vi "execute_initial_value_policy.vi"(8 "error in (no error)":errorcluster, 9 "Last Publish Time":timestamp, 10 "Last Topic Value":variant, 11 "ValueChangeSubscription In":refnum<class "ValueChangeSubscription.lvclass">) -> (0 "error out":errorcluster, 3 "ValueChangeSubscription Out":refnum<class "ValueChangeSubscription.lvclass">)   [LabVIEW 2017, in "SubscriptionPolicy.lvlib" / "ValueChangeSubscription.lvclass"]
uses:
  ValueChangeSubscription.lvclass
  ValueChangeSubscription.lvclass/ValueChangeSubscription.ctl
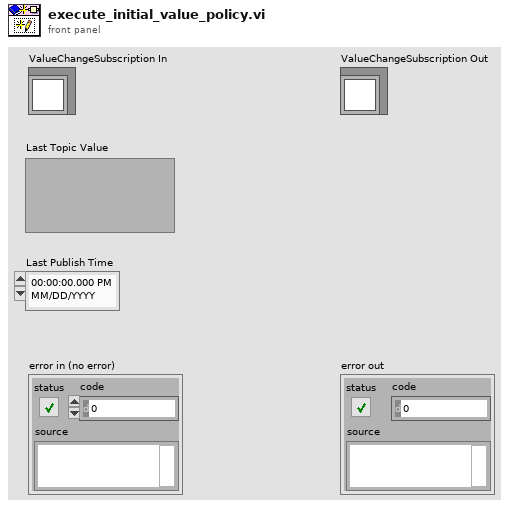
[diagram p1: front panel]
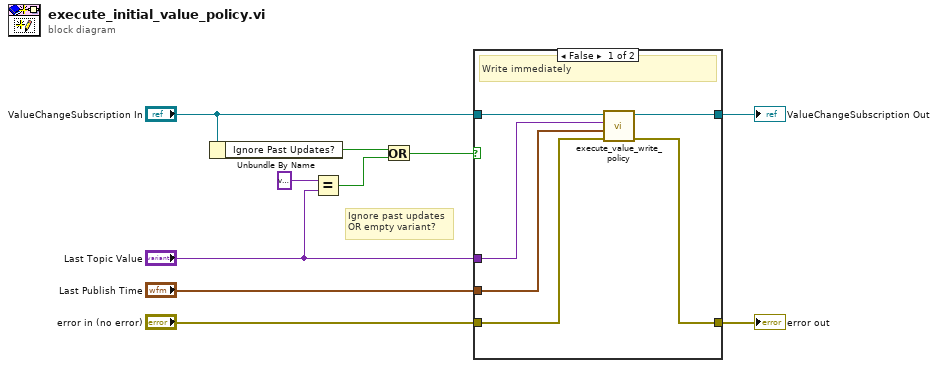
[diagram p0: block diagram]
diagram:
  # "Ignore past updates\nOR empty variant?"
  n1 = Unbundle By Name("ValueChangeSubscription In") -> ("Ignore Past Updates?"=w3:bool)
  n2 = Equal?(x=variant, y="Last Topic Value") -> (x = y?=w2:bool)
  n3 = Or(x=w3, y=w2) -> (x .or. y?=w1:bool)
  n4 = case shown="False" w1 {
    tunnel: "ValueChangeSubscription In" -> [w16 w18]
    tunnel: [w15 w18] -> w6
    tunnel: "Last Topic Value" -> [w11 _]
    tunnel: "Last Publish Time" -> [w13 _]
    tunnel: "error in (no error)" -> [w14 w17]
    tunnel: [w12 w17] -> w7
    frame False {
      # "Write immediately"
      n5 = call-dynamic "execute_value_write_policy.vi"("error in (no error)"=w14, "Publish Time"=w13, "New Topic Value"=w11, "ValueChangeSubscription In"=w16) -> ("error out"=w12:errorcluster, "ValueChangeSubscription Out"=w15:refnum<class "ValueChangeSubscription.lvclass">)  [unwired: 6 in]
    }
    frame True {
      # "Do not write immediately"
    }
  }
  "error out" <- w7
  "ValueChangeSubscription Out" <- w6
